vi "UDT_admittanceLibrary_MinimumJerkGenerateNext.vi"() -> (3 "Unit Test Framework Results":T1)   [LabVIEW 2017]
doc: "Use this template to create a user-defined test VI. Define your test requirements and wire the results to the <b>Result (Test)</b> control. Do not modify the <b>Unit Test Framework Results</b> indicator."
uses:
  <vilib>/utf/common/utf_test_result_troll.ctl
  <vilib>/utf/common/utf_test_result.ctl
  <vilib>/utf/common/utf_test_result_failure.ctl
  <vilib>/utf/common/utf_test_comparison_operators.ctl
  <vilib>/utf/common/utf_vi_tag.ctl
  RT/Admittance Controller/Controls/tf control.ctl
  RT/Admittance Controller/Controls/timer control.ctl
  RT/Admittance Controller/Controls/initial conditions control.ctl
  <vilib>/Control Software Solutions Ltd/UTF Helper/SubVIs/UTF Double Equals.vi
  RT/Admittance Controller/admittanceControllerLibrary.lvlib
  <vilib>/Control Software Solutions Ltd/UTF Helper/Unit Test Helper.lvlib
  <vilib>/utf/NI_UnitTestFramework.lvlib
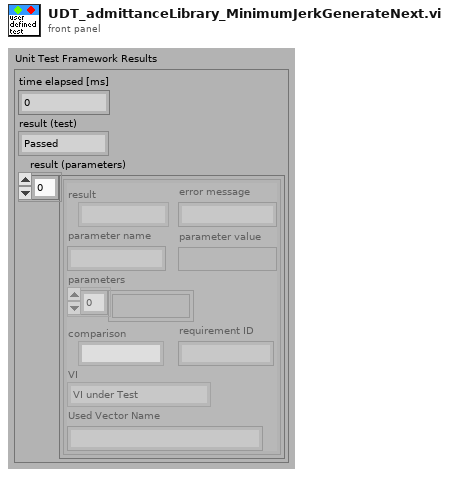
[diagram p1: front panel]
types:
  T1 = typedef "NI_UnitTestFramework.lvlib/utf_test_result_troll.ctl" = cluster{"time elapsed [ms]":u32, "result (test)":T2, "result (parameters)":T3[]}
  T2 = typedef "NI_UnitTestFramework.lvlib/utf_test_result.ctl" = enum16{"Passed", "Failed", "Error", "Skipped", "Not Processed"}
  T3 = typedef "NI_UnitTestFramework.lvlib/utf_test_result_failure.ctl" = cluster{"result":T2, "error message":string, "parameter name":string, "parameter value":variant, "parameters":variant[], "comparison":T4, "requirement ID":string, "VI":T5, "Used Vector Name":string}
  T4 = typedef "NI_UnitTestFramework.lvlib/utf_test_comparison_operators.ctl" = enum16{"=", "!=", ">", ">=", "<", "<=", "range", "symmetric tolerance", "asymmetric tolerance", "string contains", "string not contain", "array size", "string length", "array range", "by element", "array range (limit array)", "user-defined", "array contains", "array not contain", "vector length", "= (elm)", "!= (elm)", "= (case insensitive)", "!= (case insensitive)"}
  T5 = typedef "NI_UnitTestFramework.lvlib/utf_vi_tag.ctl" = enum16{"Setup VI", "VI under Test", "Teardown VI"}
  T6 = typedef "admittanceControllerLibrary.lvlib/initial conditions control.ctl" = enum16{"get", "set"}
  T7 = typedef "admittanceControllerLibrary.lvlib/timer control.ctl" = enum16{"get time", "set time"}
  T8 = typedef "admittanceControllerLibrary.lvlib/tf control.ctl" = enum16{"get tf", "set tf"}
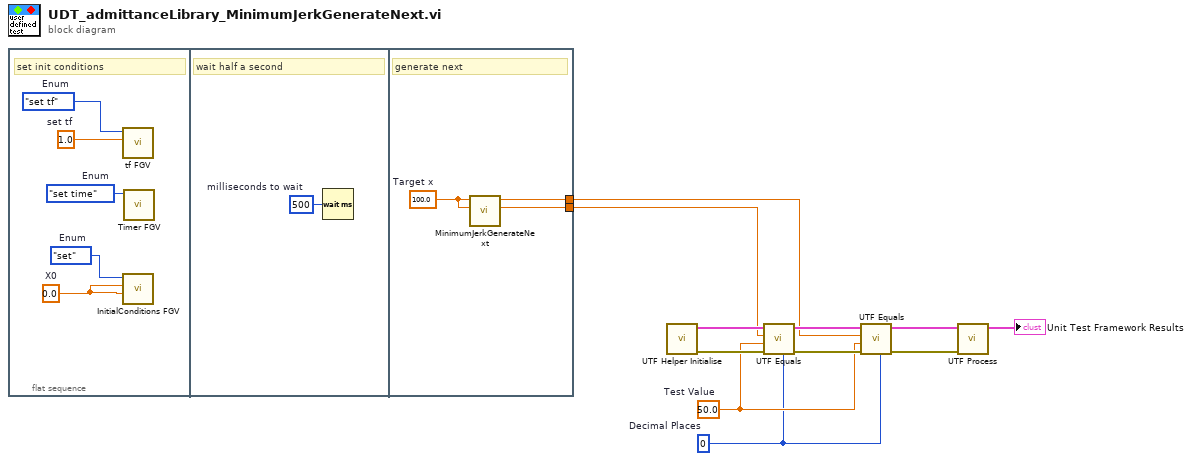
[diagram p0: block diagram]
diagram:
  w1 = u8 0  # Decimal Places
  w2 = 50.0  # Test Value
  n1 = flat-sequence {
    tunnel: [w19] -> w4
    tunnel: [w18] -> w3
    frame #0 {
      w12 = 0.0  # X0
      w13 = initial_conditions_control."set"  # Enum
      w14 = timer_control."set time"  # Enum
      w15 = 1.0  # set tf
      w16 = tf_control."set tf"  # Enum
      # "set init conditions"
      n2 = call "tf FGV.vi"("set tf"=w15, "Enum"=w16) -> ()  [unwired: 8 in, 2 out]
      n3 = call "InitialConditions FGV.vi"("Y0"=w12, "X0"=w12, "Enum"=w13) -> ()  [unwired: 6 in, 3 out]
      n4 = call "Timer FGV.vi"("Enum"=w14) -> ()  [unwired: 9 in, 2 out]
    }
    frame #1 {
      w17 = u32 500  # milliseconds to wait
      # "wait half a second"
      n5 = Wait (ms)(milliseconds to wait=w17) -> ()  [unwired: 1 out]
    }
    frame #2 {
      w20 = 100.0  # Target x
      # "generate next"
      n6 = call "MinimumJerkGenerateNext.vi"("Target y"=w20, "Target x"=w20) -> ("yt"=w19:dbl, "xt"=w18:dbl)  [unwired: 7 in, 1 out]
    }
  }
  n7 = call <vilib>:"UTF Helper Initialise.vi"() -> ("error out"=w9:errorcluster, "results array"=w10:T3[])  [unwired: 10 in]
  n8 = call-poly <vilib>:"UTF Equals.vi"("Decimal Places"=w1, "error in (no error)"=w9, "Test Value"=w2, "Input"=w4, "Input Results"=w10) -> ("error out"=w5:errorcluster, "Output Results"=w8:T3[])  [unwired: 5 in]
  n9 = call-poly <vilib>:"UTF Equals.vi"("Decimal Places"=w1, "error in (no error)"=w5, "Test Value"=w2, "Input"=w3, "Input Results"=w8) -> ("error out"=w6:errorcluster, "Output Results"=w7:T3[])  [unwired: 5 in]
  n10 = call <vilib>:"UTF Process.vi"("error in (no error)"=w6, "results array"=w7) -> ("Unit Test Framework Results"=→"Unit Test Framework Results":T1)  [unwired: 9 in]
